vi "Play One Step.vi"(0 "Display State In":T1={"method"=enum."None", "current color"=1, "available black position"=[], "available white position"=[], "Interactive Action"=refnum, "row"=0, "column"=0} caption="显示状态输入", 9 "Container State":T5 caption="容器状态", 11 "error in (no error)":errorcluster caption="错误输入（无错误）", 12 "row":i32, 13 "column":i32) -> (4 "Display State Out":T1={"method"=enum."None", "current color"=1, "available black position"=[], "available white position"=[], "Interactive Action"=refnum, "row"=0, "column"=0} caption="显示状态输出", 14 "succeed":bool, 15 "error out":errorcluster caption="错误输出")   [LabVIEW 2011, in "Othello.xctl"]
uses:
  Othello.xctl
  <vilib>/_xctls/Container State.ctl
  Ability/State.ctl
  Control/Method Call.ctl
  Control/Pict Ring Chess.ctl
  Control/Interactive Action.ctl
  <vilib>/_xctls/XControlSupport.lvlib
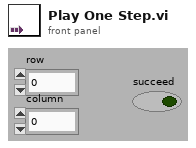
[diagram p1: front panel]
types:
  T1 = typedef "Othello.xctl/State.ctl" = cluster{"method":T2, "current color":T3, "available black position":i32[][], "available white position":i32[][], "Interactive Action":T4, "row":i32, "column":i32}
  T2 = typedef "Othello.xctl/Method Call.ctl" = enum16{"None", "New Game", "Play One"}
  T3 = typedef "Othello.xctl/Pict Ring Chess.ctl" = u16
  T4 = typedef "Othello.xctl/Interactive Action.ctl" = refnum<user-event>
  T5 = typedef "XControlSupport.lvlib/Container State.ctl" = cluster{"Indicator?":bool, "Run Mode?":bool, " Refnum":refnum<vi>}
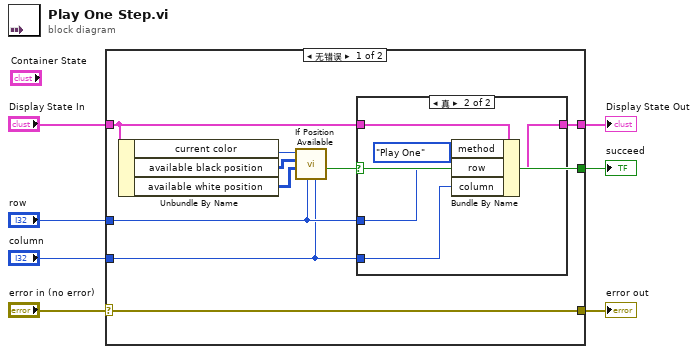
[diagram p0: block diagram]
diagram:
  n1 = case shown="无错误" "error in (no error)" {
    selector: "error in (no error)" -> [w8 w24]
    tunnel: "Display State In" -> [w16 w23]
    tunnel: [w12 _] -> w6
    tunnel: [w11 w23] -> w5
    tunnel: "row" -> [w10 _]
    tunnel: "column" -> [w9 _]
    tunnel: [w8 w24] -> w1
    frame No Error {
      n2 = Unbundle By Name(w16) -> ("current color"=w15:T3, "available black position"=w14:i32[][], "available white position"=w13:i32[][])
      n3 = call "If Position Available.vi"("column"=w9, "row"=w10, "available white position"=w13, "available black position"=w14, "current color"=w15) -> ("found?"=w12:bool)  [unwired: 6 out]
      n4 = case shown="真" w12 {
        tunnel: w16 -> [w17 w22]
        tunnel: [w17 w21] -> w11
        tunnel: w10 -> [_ w19]
        tunnel: w9 -> [_ w18]
        frame False {
        }
        frame True {
          n5 = Bundle By Name(cluster=w22, "method"=Method_Call."Play One", "row"=w19, "column"=w18) -> (w21:T1)
        }
      }
    }
    frame Error {
    }
  }
  "Display State Out" <- w5
  "error out" <- w1
  "succeed" <- w6
